vi "ModulationVoltage.vi"() -> ()   [LabVIEW 2010]
uses:
  MultiPower Meter/Global 4.vi
panel:
  in  "Current (mA)":dbl=10.0
  in  "StartFrom":i32
  out "Running":i32=10
  out "ILD(mA)":dbl
  out "PLD(mW)":dbl
  out "PLD mean":dbl
  out "ILD mean":dbl
  in  "HowLong(s)":i32
  in  "Runs":i32=10
  out "Voltage(mV)":string
  in  "FG GPIB":i16=1
  in  "Laser GPIB":u8=10 max=100
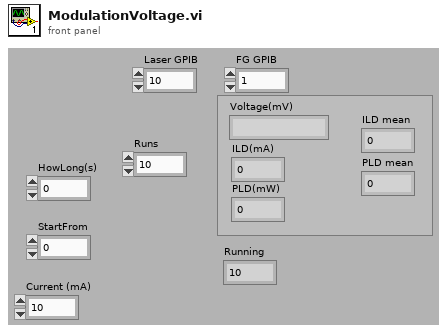
[diagram p1: front panel]
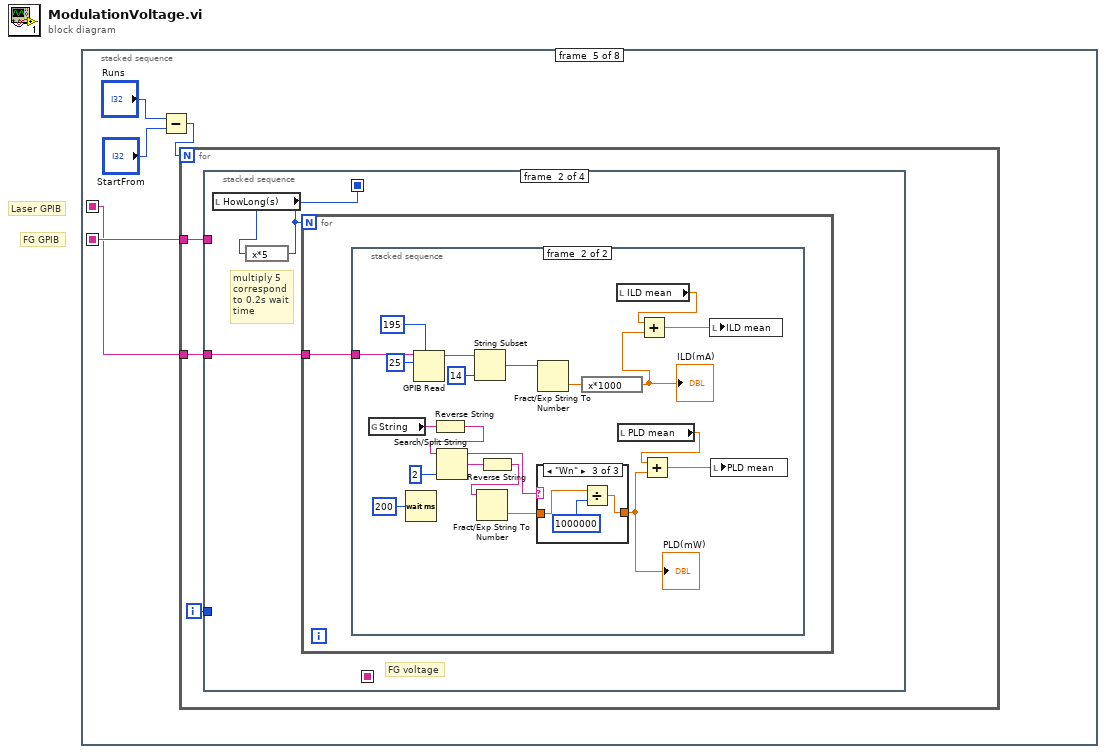
[diagram p0: block diagram]
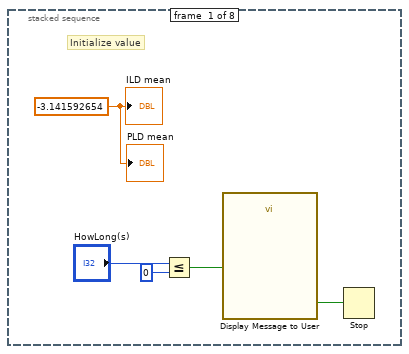
[diagram p2: hidden frame]
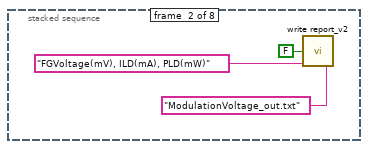
[diagram p3: hidden frame]
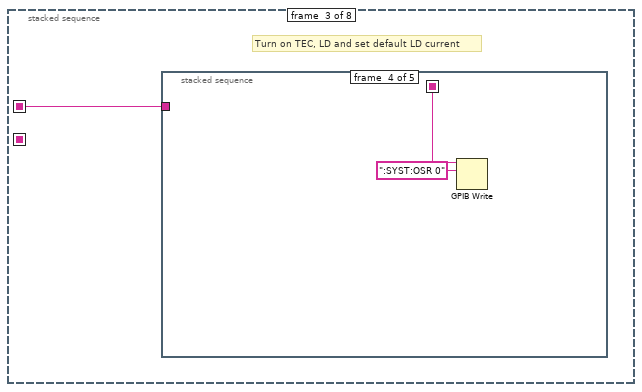
[diagram p4: hidden frame]
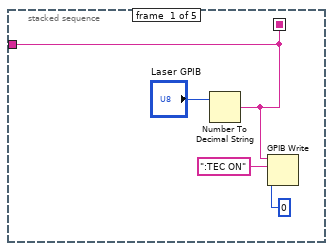
[diagram p5: hidden frame]
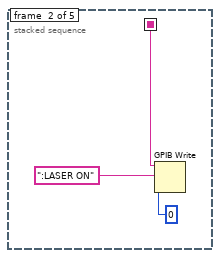
[diagram p6: hidden frame]
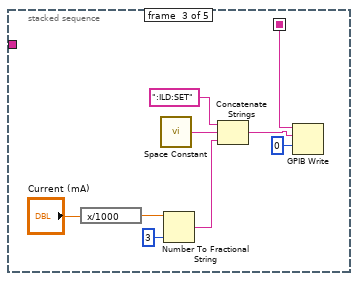
[diagram p7: hidden frame]
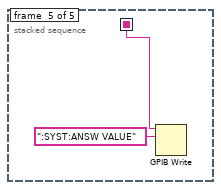
[diagram p8: hidden frame]
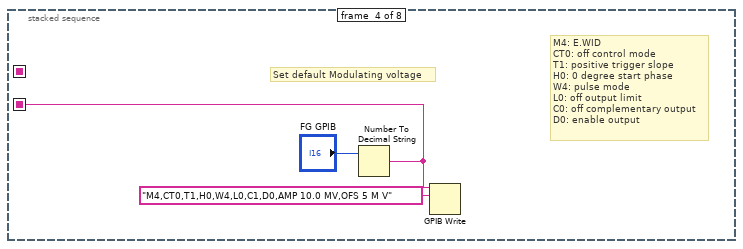
[diagram p9: hidden frame]
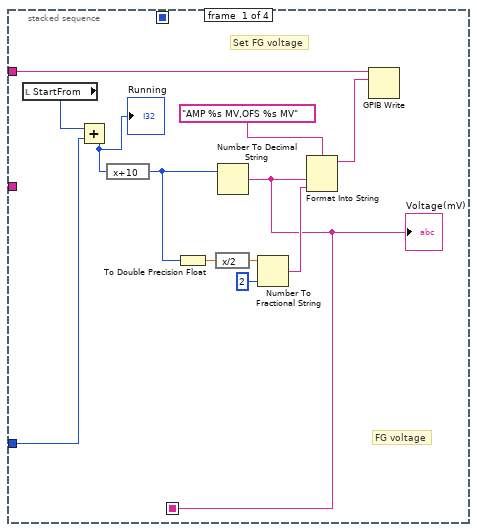
[diagram p10: hidden frame]
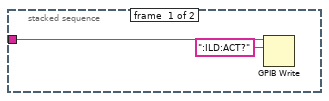
[diagram p11: hidden frame]
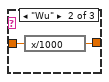
[diagram p13: hidden frame]
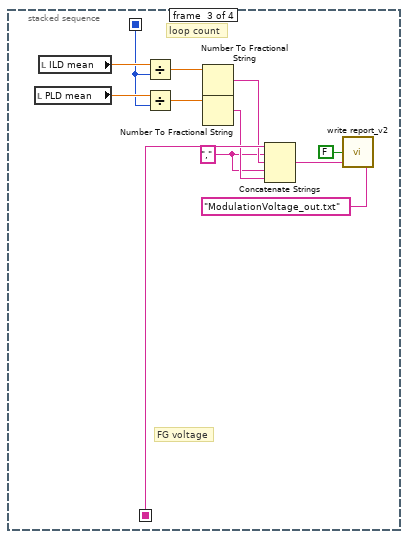
[diagram p14: hidden frame]
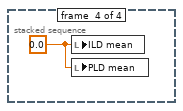
[diagram p15: hidden frame]
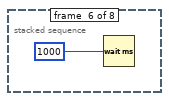
[diagram p16: hidden frame]
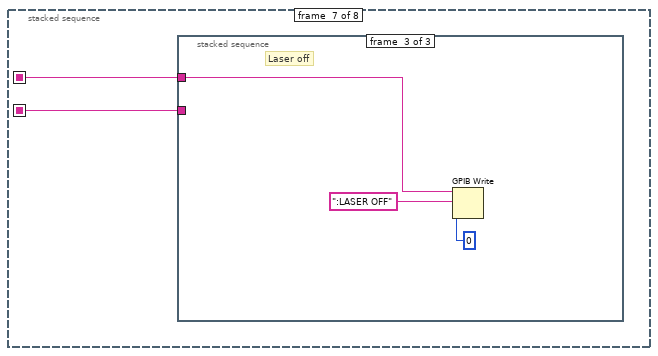
[diagram p17: hidden frame]
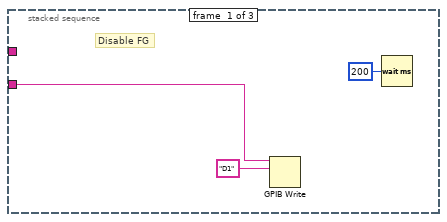
[diagram p18: hidden frame]
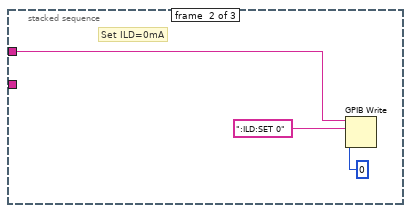
[diagram p19: hidden frame]
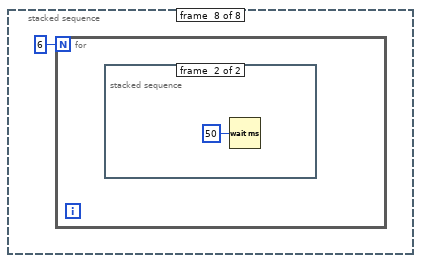
[diagram p20: hidden frame]
diagram:
  # "FG GPIB"
  # "Laser GPIB"
  n1 = stacked-sequence {
    seq-local: [_ _ w9 _ _ _ _ _] -> [_ _ _ _ w36 _ w101 _]
    seq-local: [_ _ _ w30 _ _ _ _] -> [_ _ _ _ w37 _ w100 _]
    frame #0 {
      w5 = -3.141592654 ("ILD mean")
      # "Initialize value"
      n2 = Less Or Equal?(x="HowLong(s)", y=0) -> (x <= y?=w2:bool)
      n3 = call "Display Message to User"("Enable"=w2) -> ("OK"=w1:bool)  [unwired: 9 in, 1 out]
      n4 = Stop(stop? (T)=w1) -> ()
      "ILD mean" <- w5
      "PLD mean" <- w5
    }
    frame #1 {
      n5 = call "write report_v2.vi"("fixed filename"="ModulationVoltage_out.txt" ("filename"), "input"="FGVoltage(mV), ILD(mA), PLD(mW)" ("string"), "Multiple File?"=FALSE) -> ()  [unwired: 2 in]
    }
    frame #2 {
      # "Turn on TEC, LD and set default LD current"
      n6 = stacked-sequence {
        seq-local: [w10 _ _ _ _] -> [_ w14 w24 w27 w28]
        tunnel: [w10 _ _ _ _] -> w9
        frame #0 {
          n7 = Number To Decimal String(number="Laser GPIB") -> (decimal integer string=w10:string)  [unwired: 1 in]
          n8 = GPIB Write(0:w10, 1:":TEC ON" ("data"), 2:i16 0 ("mode (0)")) -> ()  [unwired: 2 in, 2 out]
        }
        frame #1 {
          n9 = GPIB Write(0:w14, 1:":LASER ON" ("data"), 2:i16 0 ("mode (0)")) -> ()  [unwired: 2 in, 2 out]
        }
        frame #2 {
          n10 = expression code="x/1000"("Current (mA)") -> (w20:dbl)
          n11 = call <vilib>:"Space Constant.vi"() -> ("String"=w19:string)
          n12 = Number To Fractional String(number=w20, precision (6)=i16 3) -> (F-format string=w23:string)  [unwired: 2 in]
          n13 = Concatenate Strings(":ILD:SET", w19, w23) -> (w17:string)
          n14 = GPIB Write(0:w24, 1:w17, 2:i16 0 ("mode (0)")) -> ()  [unwired: 2 in, 2 out]
        }
        frame #3 {
          n15 = GPIB Write(0:w27, 1:":SYST:OSR 0" ("data")) -> ()  [unwired: 3 in, 2 out]
        }
        frame #4 {
          n16 = GPIB Write(0:w28, 1:":SYST:ANSW VALUE" ("data")) -> ()  [unwired: 3 in, 2 out]
        }
      }
    }
    frame #3 {
      # "M4: E.WID\nCT0: off control mode\nT1: positive trigger slope\nH0: 0 degree start phase\nW4: pulse mode\nL0: off output limit\nC0: off complementary output\nD0: enable output"
      # "Set default Modulating voltage"
      n17 = Number To Decimal String(number="FG GPIB") -> (decimal integer string=w30:string)  [unwired: 1 in]
      n18 = GPIB Write(0:w30, 1:"M4,CT0,T1,H0,W4,L0,C1,D0,AMP 10.0 MV,OFS 5 M V") -> ()  [unwired: 3 in, 2 out]
    }
    frame #4 {
      n19 = Subtract(x="Runs", y="StartFrom") -> (x-y=w33:i32)
      n20 = for {
        N: w33 -> [_]
        tunnel: w37 -> [w40]
        tunnel: w36 -> [w38]
        i -> [w39]
        n21 = stacked-sequence {
          seq-local: [w45 _ _ _] -> [_ _ w92 _]
          seq-local: [_ w54 _ _] -> [_ _ w95 _]
          tunnel: w40 -> [w52 _ _ _]
          tunnel: w39 -> [w43 _ _ _]
          tunnel: w38 -> [_ w55 _ _]
          frame #0 {
            # "FG voltage"
            # "Set FG voltage"
            n22 = local read "StartFrom"() -> (w41:i32)
            n23 = Add(x=w41, y=w43) -> (x+y=w42:i32)
            "Running" <- w42
            n24 = expression code="x+10"(w42) -> (w44:i32)
            n25 = To Double Precision Float(number=w44) -> (double precision float=w50:dbl)
            n26 = expression code="x/2"(w50) -> (w49:dbl)
            n27 = Number To Decimal String(number=w44) -> (decimal integer string=w45:string)  [unwired: 1 in]
            "Voltage(mV)" <- w45
            n28 = Number To Fractional String(number=w49, precision (6)=i16 2) -> (F-format string=w48:string)  [unwired: 2 in]
            n29 = Format Into String(format string="AMP %s MV,OFS %s MV", w45, w48) -> (resulting string=w47:string)  [unwired: 2 in, 1 out]
            n30 = GPIB Write(0:w52, 1:w47) -> ()  [unwired: 3 in, 2 out]
          }
          frame #1 {
            # "FG voltage"
            # "multiply 5 \ncorrespond\nto 0.2s wait\ntime"
            n31 = local read "HowLong(s)"() -> (w53:i32)
            n32 = expression code="x*5"(w53) -> (w54:i32)
            n33 = for {
              N: w54 -> [_]
              tunnel: w55 -> [w56]
              n34 = stacked-sequence {
                tunnel: w56 -> [w58 w79]
                frame #0 {
                  n35 = GPIB Write(0:w58, 1:":ILD:ACT?" ("data")) -> ()  [unwired: 3 in, 2 out]
                }
                frame #1 {
                  n36 = global read "Global 4.vi" "String"() -> (w65:string)
                  n37 = Wait (ms)(milliseconds to wait=u32 200) -> ()  [unwired: 1 out]
                  n38 = GPIB Read(0:w79, 1:25 ("byte count"), 4:195 ("timeout ms (488.2 global)")) -> (5:w75:string)  [unwired: 2 in, 2 out]
                  n39 = Reverse String(1:w65) -> (0:w68:string)
                  n40 = Search/Split String(string=w68, offset (0)=2) -> (substring before match=w63:string, match + rest of string=w66:string)  [unwired: 1 in, 1 out]
                  n41 = String Subset(string=w75, length (rest)=14 ("length (rest)")) -> (substring=w73:string)  [unwired: 1 in]
                  n42 = Reverse String(1:w66) -> (0:w64:string)
                  n43 = Fract/Exp String To Number(string=w64) -> (number=w62:dbl)  [unwired: 3 in, 1 out]
                  n44 = case shown="\"Wn\"" w63 {
                    tunnel: [w80 w81 w85] -> w61
                    tunnel: w62 -> [w80 w82 w84]
                    frame "Wm", Default {
                    }
                    frame "Wu" {
                      n45 = expression code="x/1000"(w82) -> (w81:dbl)
                    }
                    frame "Wn" {
                      n46 = Divide(x=w84, y=1000000) -> (x/y=w85:dbl)
                    }
                  }
                  "PLD(mW)" <- w61
                  n47 = Fract/Exp String To Number(string=w73) -> (number=w60:dbl)  [unwired: 3 in, 1 out]
                  n48 = expression code="x*1000"(w60) -> (w59:dbl)
                  "ILD(mA)" <- w59
                  n49 = local read "ILD mean"() -> (w72:dbl)
                  n50 = local read "PLD mean"() -> (w69:dbl)
                  n51 = Add(x=w72, y=w59) -> (x+y=w71:dbl)
                  n52 = Add(x=w69, y=w61) -> (x+y=w70:dbl)
                  n53 = local write "ILD mean"(w71) -> ()
                  n54 = local write "PLD mean"(w70) -> ()
                }
              }
            }
          }
          frame #2 {
            w89 = "," ("string")
            # "loop count"
            # "FG voltage"
            n55 = local read "PLD mean"() -> (w96:dbl)
            n56 = local read "ILD mean"() -> (w97:dbl)
            n57 = Divide(x=w97, y=w95) -> (x/y=w94:dbl)
            n58 = Divide(x=w96, y=w95) -> (x/y=w93:dbl)
            n59 = Number To Fractional String(number=w94) -> (F-format string=w91:string)  [unwired: 3 in]
            n60 = Number To Fractional String(number=w93) -> (F-format string=w90:string)  [unwired: 3 in]
            n61 = Concatenate Strings(w92, w89, w91, w89, w90) -> (w88:string)
            n62 = call "write report_v2.vi"("fixed filename"="ModulationVoltage_out.txt" ("filename"), "input"=w88, "Multiple File?"=FALSE) -> ()  [unwired: 2 in]
          }
          frame #3 {
            w98 = 0.0 ("ILD mean")
            n63 = local write "ILD mean"(w98) -> ()
            n64 = local write "PLD mean"(w98) -> ()
          }
        }
      }
    }
    frame #5 {
      n65 = Wait (ms)(milliseconds to wait=u32 1000 ("Wait after finish")) -> ()  [unwired: 1 out]
    }
    frame #6 {
      n66 = stacked-sequence {
        tunnel: w101 -> [_ w106 w108]
        tunnel: w100 -> [w103 _ _]
        frame #0 {
          # "Disable FG"
          n67 = GPIB Write(0:w103, 1:"D1") -> ()  [unwired: 3 in, 2 out]
          n68 = Wait (ms)(milliseconds to wait=u32 200) -> ()  [unwired: 1 out]
        }
        frame #1 {
          # "Set ILD=0mA"
          n69 = GPIB Write(0:w106, 1:":ILD:SET 0", 2:i16 0 ("mode (0)")) -> ()  [unwired: 2 in, 2 out]
        }
        frame #2 {
          # "Laser off"
          n70 = GPIB Write(0:w108, 1:":LASER OFF" ("data"), 2:i16 0 ("mode (0)")) -> ()  [unwired: 2 in, 2 out]
        }
      }
    }
    frame #7 {
      n71 = for {
        N: 6 -> [_]
        n72 = stacked-sequence {
          frame #0 {
            n73 = call <vilib>:"Beep.vi"("use system alert? (T)"=FALSE, "duration (msec)"=u32 100, "frequency (Hz)"=u32 700) -> ()  [unwired: 9 in]
          }
          frame #1 {
            n74 = Wait (ms)(milliseconds to wait=u32 50) -> ()  [unwired: 1 out]
          }
        }
      }
    }
  }
